vi "UI_ShowIn_Subpanel.vi"(8 "error in (no error)":errorcluster, 10 "Sub Panel":refnum<vi>, 11 "UI_Actor in":refnum<class "UI_Actor.lvclass">) -> (0 "error out":errorcluster, 3 "UI_Actor out":refnum<class "UI_Actor.lvclass">)   [LabVIEW 2020, in "UI_Actor.lvlib" / "UI_Actor.lvclass"]
uses:
  UI_Actor.lvclass
  UI_Actor.lvclass/UI_Actor.ctl
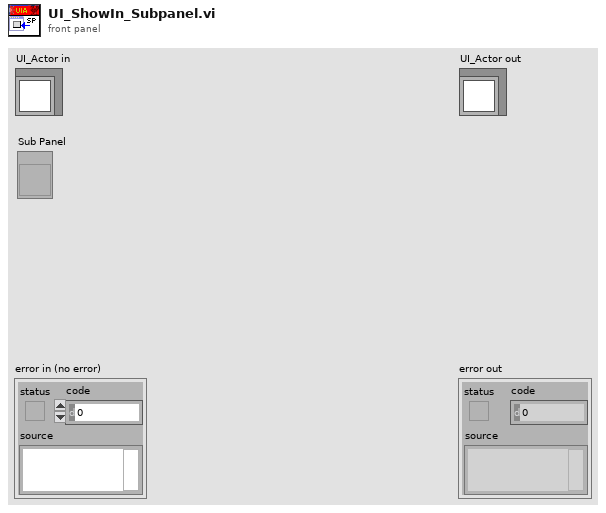
[diagram p1: front panel]
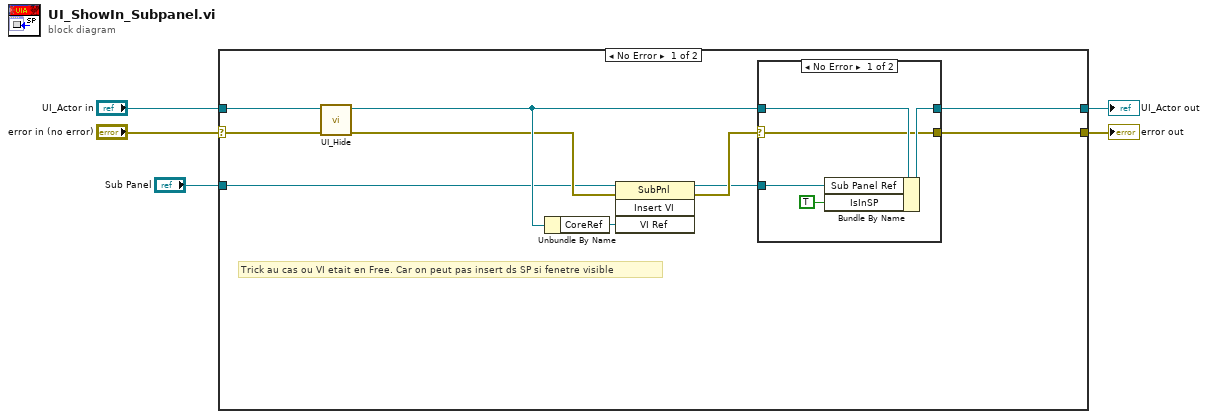
[diagram p0: block diagram]
diagram:
  n1 = case shown="No Error" "error in (no error)" {
    selector: "error in (no error)" -> [w13 w24]
    tunnel: [w8 w24] -> w4
    tunnel: [w9 w23] -> w2
    tunnel: "UI_Actor in" -> [w14 w23]
    tunnel: "Sub Panel" -> [w7 _]
    frame No Error {
      # "Trick au cas ou VI etait en Free. Car on peut pas insert ds SP si fenetre visible"
      n2 = call-dynamic "UI_Hide.vi"("error in (no error)"=w13, "UI_Actor in"=w14) -> ("error out"=w11:errorcluster, "UI_Actor out"=w12:refnum<class "UI_Actor.lvclass">)  [unwired: 8 in]
      n3 = Unbundle By Name(w12) -> ("CoreRef"=w15:refnum<vi>)
      n4 = invoke class="SubPnl" method="Insert VI"(reference=w7, error in=w11, "VI Ref"=w15) -> (reference out=w6:refnum<vi>, error out=w10:errorcluster)  [unwired: 1 in, 2 out]
      n5 = case shown="No Error" w10 {
        selector: w10 -> [w18 w21]
        tunnel: [w19 w22] -> w9
        tunnel: w12 -> [w20 w22]
        tunnel: [w18 w21] -> w8
        tunnel: w6 -> [w17 _]
        frame No Error {
          n6 = Bundle By Name(cluster=w20, "Sub Panel Ref"=w17, "IsInSP"=TRUE ("Window management.IsInSP")) -> (w19:refnum<class "UI_Actor.lvclass">)
        }
        frame Error {
        }
      }
    }
    frame Error {
    }
  }
  "error out" <- w4
  "UI_Actor out" <- w2
